vi "Stall A arm Raise.vi"(7 "Port (Port A)":T1 items=["Port A", "Port B", "Port C", "Port D"], 9 "Power":i8=90, 11 "NXT/EV3":T2) -> (3 "NXT/EV3":T2)   [LabVIEW 2016]
uses:
  <vilib>/NXT/Subs/LVHSConnector.ctl
  <vilib>/NXT/LegoClasses/BrickReference/BrickReference.lvclass
  <vilib>/NXT/Block Support/NXT_OutputPort.ctl
  <vilib>/NXT/Block Support/NXT_TimerIndex.ctl
  <vilib>/NXT/NXTIO Xnodes/NXTIONodeSubVIs/NXTMoveMotors.vi
  <vilib>/NXT/NXTIO Xnodes/NXTIONodeSubVIs/LEGOResetMotors.vi
  <vilib>/NXT/Dual Mode Library/Sensors/Reset_Timer.vi
  <vilib>/NXT/Dual Mode Library/Waits/Wait_Num.vi
  <vilib>/NXT/Dual Mode Library/Motors/Rotation.vi
  <vilib>/NXT/Dual Mode Library/Sensors/Read_Timer.vi
  <vilib>/NXT/NXTIO Xnodes/NXTIONodeSubVIs/NXTStopMotors.vi
  <vilib>/NXT/NXTIO Xnodes/NXTIOXNode/NXTIO.xnode
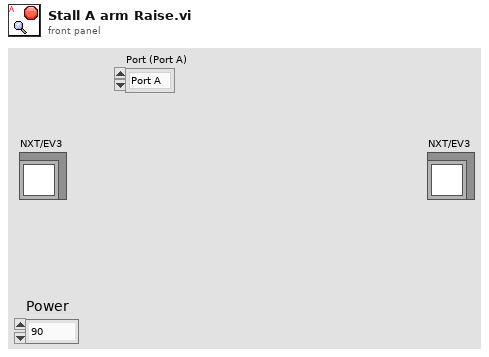
[diagram p1: front panel]
types:
  T1 = typedef "NXT_OutputPort.ctl" = u8
  T2 = typedef "LVHSConnector.ctl" = refnum<class "BrickReference.lvclass">
  T3 = typedef "NXT_TimerIndex.ctl" = u8
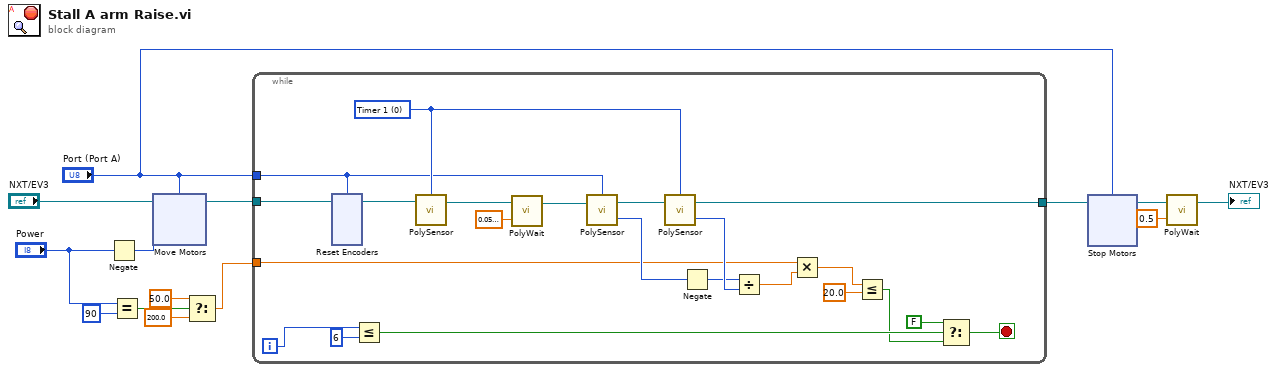
[diagram p0: block diagram]
diagram:
  n1 = Negate(x="Power") -> (-x=w7:i8)
  n2 = Equal?(x="Power", y=i8 90) -> (x = y?=w4:bool)
  n3 = xnode "Move Motors"("Power/Speed 1"=w7, "Motors"="Port (Port A)", "NXT/EV3"="NXT/EV3") -> ("NXT/EV3"=w14:T2)
  n4 = Select(t=50.0, s=w4, f=200.0) -> (s? t:f=w1:dbl)
  n5 = while {
    tunnel: w14 -> [w28]
    tunnel: [w27] -> w13
    tunnel: "Port (Port A)" -> [w26]
    tunnel: w1 -> [w17]
    i -> [w16]
    stop <- w20 stop-if-true
    w32 = T3 0 items=["Timer 1", "Timer 2", "Timer 3"] ("Timer (Timer 1)")
    n6 = xnode "Reset Encoders"("Motors"=w26, "NXT/EV3"=w28) -> ("NXT/EV3"=w36:T2)
    n7 = Less Or Equal?(x=w16, y=6) -> (x <= y?=w22:bool)
    n8 = call-poly <vilib>:"PolySensor.vi"("NXT/EV3"=w36, "Timer (Timer 1)"=w32) -> ("NXT/EV3"=w35:T2)  [unwired: 2 in]
    n9 = call-poly <vilib>:"PolyWait.vi"("Time (1 sec)"=sgl 0.05, "NXT/EV3"=w35) -> ("NXT/EV3"=w33:T2)  [unwired: 2 in]
    n10 = call-poly <vilib>:"PolySensor.vi"("NXT/EV3"=w33, "Port (Port A)"=w26) -> ("Angle of Rotation"=w30:i32, "NXT/EV3"=w31:T2)  [unwired: 1 in]
    n11 = call-poly <vilib>:"PolySensor.vi"("NXT/EV3"=w31, "Timer (Timer 1)"=w32) -> ("Value (msec)"=w29:u32, "NXT/EV3"=w27:T2)  [unwired: 1 in]
    n12 = Negate(x=w30) -> (-x=w18:i32)
    n13 = Divide(x=w18, y=w29) -> (x/y=w25:dbl)
    n14 = Multiply(x=w17, y=w25) -> (x*y=w24:dbl)
    n15 = Less Or Equal?(x=w24, y=20.0) -> (x <= y?=w19:bool)
    n16 = Select(t=FALSE, s=w22, f=w19) -> (s? t:f=w20:bool)
  }
  n17 = xnode "Stop Motors"("Motors"="Port (Port A)", "NXT/EV3"=w13) -> ("NXT/EV3"=w10:T2)
  n18 = call-poly <vilib>:"PolyWait.vi"("Time (1 sec)"=sgl 0.5, "NXT/EV3"=w10) -> ("NXT/EV3"=→"NXT/EV3":T2)  [unwired: 2 in]
